vi "rs3_cull_points.vi"(11 "input vertices":dbl[][](array[numeric])=array32964x6[197784 elements]) -> (1 "Valid vertices":bool[](array[boolean]), 2 "output valid vertices":dbl[][](array[numeric]), 3 "Output vertices":string[][](array[string]))   [LabVIEW 2017, in "libRealSense3.lvlib"]
uses:
  libRealSense3.lvlib
panel:
  out "Array 3":bool[](array[boolean])=[FALSE, TRUE, FALSE, TRUE, FALSE, TRUE, FALSE, TRUE, FALSE, TRUE, FALSE, TRUE, FALSE, TRUE, FALSE, TRUE, FALSE, TRUE, FALSE, TRUE, FALSE, TRUE, FALSE, TRUE, FALSE, TRUE, FALSE, TRUE, FALSE, TRUE, FALSE, TRUE, FALSE, TRUE, FALSE, TRUE, FALSE, TRUE, FALSE, TRUE, FALSE, TRUE, FALSE, TRUE, FALSE, TRUE, FALSE, TRUE, FALSE, TRUE, FALSE, TRUE, FALSE, TRUE, FALSE, TRUE, FALSE, TRUE, FALSE, TRUE, FALSE, TRUE, FALSE, TRUE, FALSE, TRUE, FALSE, TRUE, FALSE, TRUE, FALSE, TRUE, FALSE, TRUE, FALSE, TRUE, FALSE, TRUE, FALSE, TRUE, FALSE, TRUE, FALSE, TRUE, FALSE, TRUE, FALSE, TRUE, FALSE, TRUE, FALSE, TRUE, FALSE, TRUE, FALSE, TRUE, FALSE, TRUE, FALSE, TRUE, FALSE, TRUE, FALSE, TRUE, FALSE, TRUE, FALSE, TRUE, FALSE, TRUE, FALSE, TRUE, FALSE, TRUE, FALSE, TRUE, FALSE, TRUE, FALSE, TRUE, FALSE, TRUE, FALSE, TRUE, FALSE, TRUE, FALSE, TRUE, FALSE, TRUE, FALSE, TRUE, FALSE, TRUE, FALSE, TRUE, FALSE, TRUE, FALSE, TRUE, FALSE, TRUE, FALSE, TRUE, FALSE, TRUE, FALSE, TRUE, FALSE, TRUE, FALSE, TRUE, FALSE, TRUE, FALSE, TRUE, FALSE, TRUE, FALSE, TRUE, FALSE, TRUE, FALSE, TRUE, FALSE, TRUE, FALSE, TRUE, FALSE, TRUE, FALSE, TRUE, FALSE, TRUE, FALSE, TRUE, FALSE, TRUE, FALSE, TRUE, FALSE, TRUE, FALSE, TRUE, FALSE, TRUE, FALSE, TRUE, FALSE, TRUE, FALSE, TRUE, FALSE, TRUE, FALSE, TRUE, FALSE, TRUE, FALSE, TRUE, FALSE, TRUE, FALSE, TRUE, FALSE, TRUE, FALSE, TRUE, FALSE, TRUE, FALSE, TRUE, FALSE, TRUE, FALSE, TRUE, FALSE, TRUE, FALSE, TRUE, FALSE, TRUE, FALSE, TRUE, FALSE, TRUE, FALSE, TRUE, FALSE, TRUE, FALSE, TRUE, FALSE, TRUE, FALSE, TRUE, FALSE, TRUE, FALSE, TRUE, FALSE, TRUE, FALSE, TRUE, FALSE, TRUE, FALSE, TRUE, FALSE, TRUE, FALSE, TRUE, FALSE, TRUE, FALSE, TRUE, FALSE, TRUE, FALSE, TRUE, FALSE, TRUE, FALSE, TRUE, FALSE, TRUE, FALSE, TRUE, FALSE, TRUE, FALSE, TRUE, FALSE, TRUE, FALSE, TRUE, FALSE, TRUE, FALSE, TRUE, FALSE, TRUE, FALSE, TRUE, FALSE, TRUE, FALSE, TRUE, FALSE, TRUE, FALSE, TRUE, FALSE, TRUE, FALSE, TRUE, FALSE, TRUE, FALSE, TRUE, FALSE, TRUE, FALSE, TRUE, FALSE, TRUE, FALSE, TRUE, FALSE, TRUE, FALSE, TRUE, FALSE, TRUE, FALSE, TRUE, FALSE, TRUE, FALSE, TRUE, FALSE, TRUE, FALSE, TRUE, FALSE, TRUE, FALSE, TRUE, FALSE, TRUE, FALSE, TRUE, FALSE, TRUE, FALSE, TRUE, FALSE, TRUE, FALSE, TRUE, FALSE, TRUE, FALSE, TRUE, FALSE, TRUE, FALSE, TRUE, FALSE, TRUE, FALSE, TRUE, FALSE, TRUE, FALSE, TRUE, FALSE, TRUE, FALSE, TRUE, FALSE, TRUE, FALSE, TRUE, FALSE, TRUE, FALSE, TRUE, FALSE, TRUE, FALSE, TRUE, FALSE, TRUE, FALSE, TRUE, FALSE, TRUE, FALSE, TRUE, FALSE, TRUE, FALSE, TRUE, FALSE, TRUE, FALSE, TRUE, FALSE, TRUE, FALSE, TRUE, FALSE, TRUE, FALSE, TRUE, FALSE, TRUE, FALSE, TRUE, FALSE, TRUE]
  out "last size":i32=134
  out "last valid":bool=TRUE
  out "Array 2":i32[](array[numeric])=[32, 132, 33, 131, 33, 131, 33, 131, 34, 130, 35, 129, 35, 129, 36, 128, 36, 128, 35, 129, 37, 127, 37, 127, 38, 126, 38, 126, 35, 129, 34, 130, 34, 130, 34, 130, 34, 130, 34, 130, 34, 130, 34, 130, 34, 130, 34, 130, 35, 129, 36, 128, 37, 127, 37, 127, 36, 128, 35, 129, 35, 129, 34, 130, 34, 130, 34, 130, 34, 130, 34, 130, 34, 130, 33, 131, 33, 131, 33, 131, 33, 131, 33, 131, 33, 131, 32, 132, 33, 131, 34, 130, 34, 130, 34, 130, 34, 130, 33, 131, 33, 131, 33, 131, 33, 131, 32, 132, 32, 132, 32, 132, 32, 132, 32, 132, 32, 132, 32, 132, 33, 131, 32, 132, 31, 133, 31, 133, 32, 132, 31, 133, 32, 132, 32, 132, 32, 132, 32, 132, 32, 132, 32, 132, 33, 131, 34, 130, 35, 129, 35, 129, 35, 129, 33, 131, 33, 131, 33, 131, 33, 131, 33, 131, 32, 132, 32, 132, 32, 132, 32, 132, 32, 132, 32, 132, 32, 132, 33, 131, 34, 130, 35, 129, 35, 129, 35, 129, 35, 129, 35, 129, 34, 130, 34, 130, 33, 131, 33, 131, 34, 130, 33, 131, 34, 130, 34, 130, 34, 130, 33, 131, 32, 132, 33, 131, 33, 131, 34, 130, 34, 130, 34, 130, 34, 130, 33, 131, 33, 131, 33, 131, 32, 132, 32, 132, 31, 133, 30, 134, 31, 133, 31, 133, 31, 133, 31, 133, 31, 133, 32, 132, 32, 132, 33, 131, 33, 131, 33, 131, 32, 132, 31, 133, 31, 133, 31, 133, 31, 133, 30, 134, 30, 134, 29, 135, 29, 135, 30, 134, 30, 134, 30, 134, 31, 133, 31, 133, 31, 133, 31, 133, 32, 132, 32, 132, 32, 132, 34, 130, 34, 130, 32, 132, 32, 132, 31, 133, 31, 133, 31, 133, 32, 132, 31, 133, 31, 133, 31, 133, 31, 133, 30, 134, 30, 134, 31, 133, 31, 133, 31, 133, 31, 133, 31, 133, 31, 133, 31, 133, 32, 132, 30, 134, 30, 134, 30, 134, 30, 134, 31, 133, 31, 133, 31, 133, 31, 133, 31, 133, 31, 133, 31, 133, 32, 132, 33, 131, 33, 131, 33, 131, 33, 131, 33, 131, 34, 130, 34, 130, 33, 131, 32, 132, 32, 132, 32, 132, 31, 133, 31, 133, 32, 132, 32, 132, 31, 133, 30, 134, 30, 134]
  out "size(s)":i32[](array[numeric])=[32964, 6]
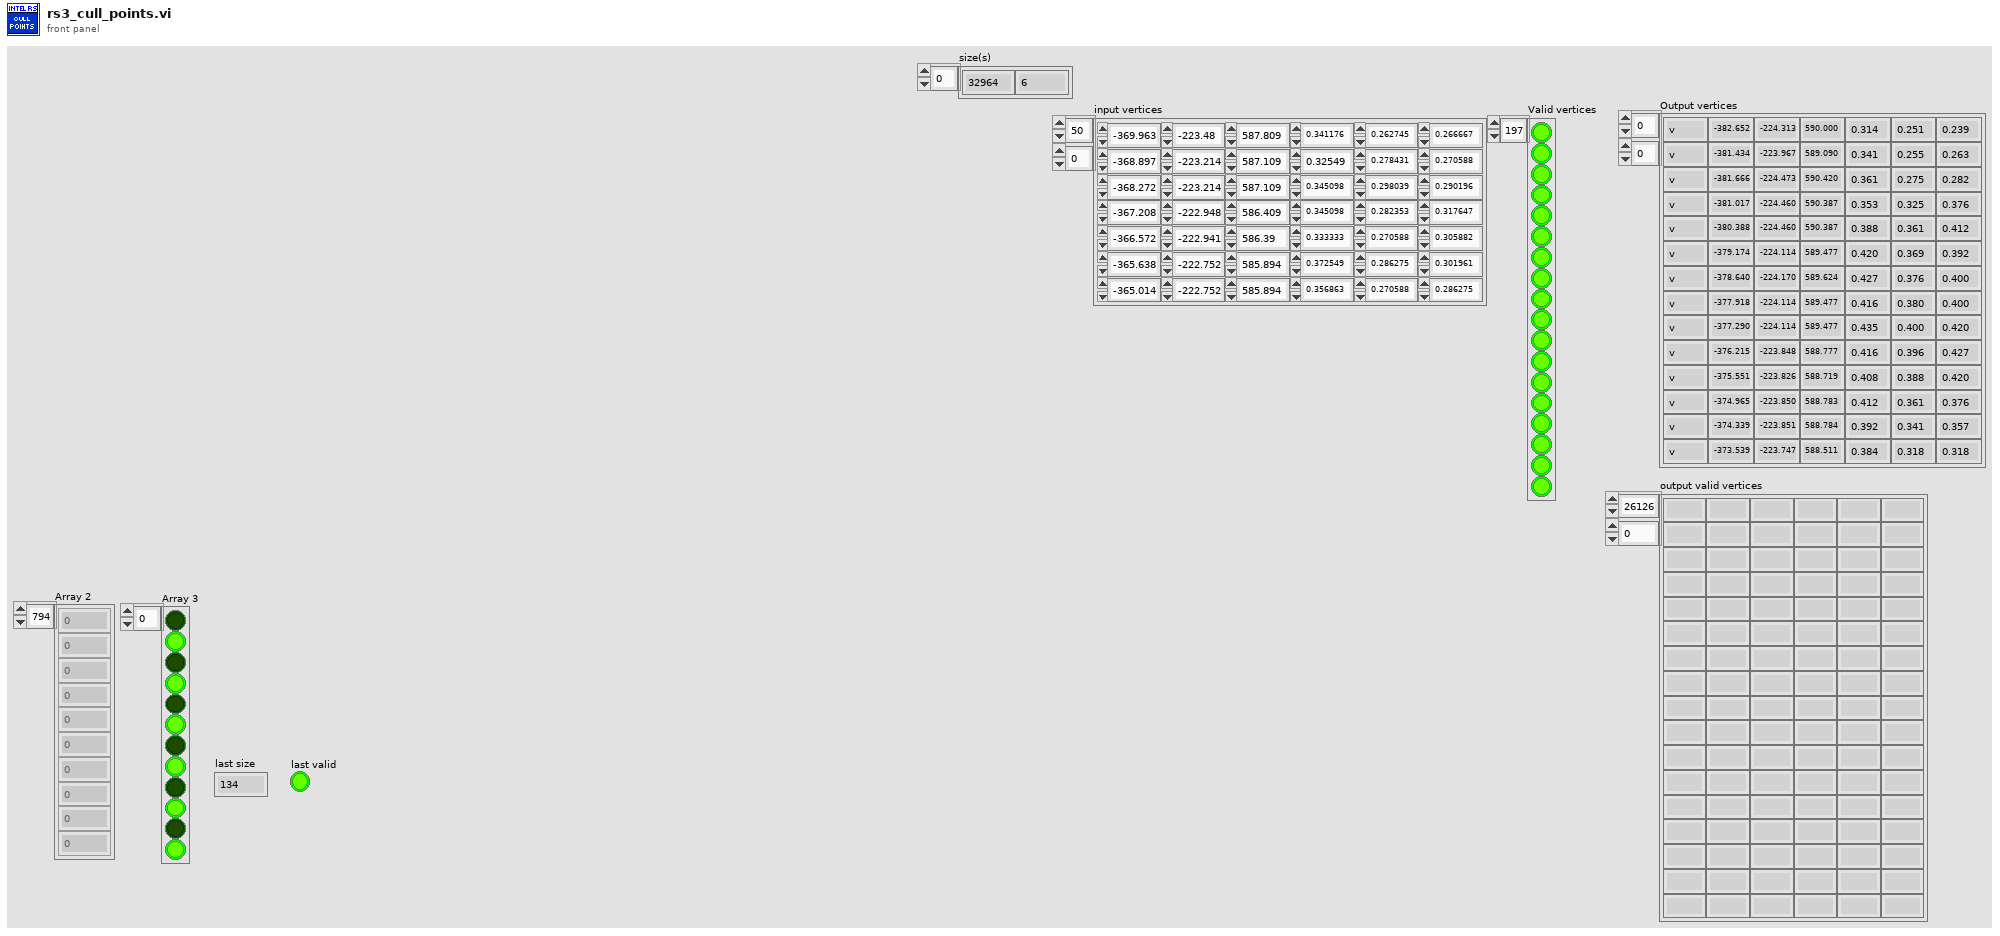
[diagram p1: front panel]
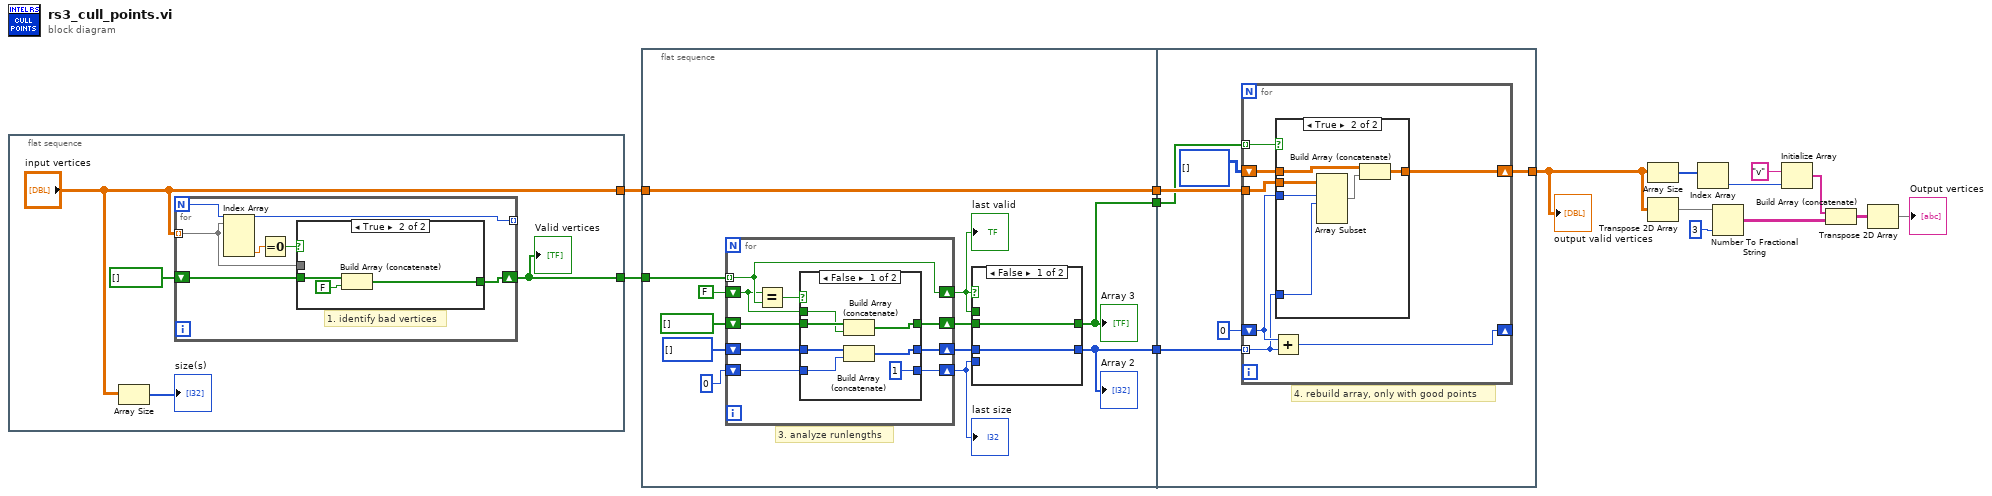
[diagram p0: block diagram]
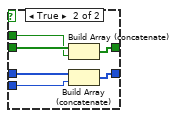
[diagram p2: hidden frame]
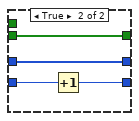
[diagram p3: hidden frame]
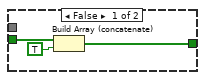
[diagram p5: hidden frame]
diagram:
  n1 = flat-sequence {
    tunnel: [w17] -> w1
    tunnel: ["input vertices"] -> w2
    frame #0 {
      n2 = Array Size(array="input vertices") -> (size(s)=→"size(s)":i32[])
      n3 = for {
        N -> [w23]
        tunnel: "input vertices" -> [w25] mode=indexing
        tunnel: [w23] -> _ mode=indexing
        shift-right: [w21] -> w17
        shift-left: bool[] [] -> [w22]
        # "1. identify bad vertices"
        n4 = Index Array(array=w25) -> (element #3=w20:dbl)  [unwired: 3 in, 2 out]
        n5 = Equal To 0?(x=w20) -> (x = 0?=w24:bool)
        n6 = case shown="True" w24 {
          tunnel: w25 -> [_ _]
          tunnel: [w28 w29] -> w21
          tunnel: w22 -> [w26 w31]
          frame False {
            n7 = Build Array (concatenate)(w26, TRUE) -> (w28:bool[])
          }
          frame True {
            n8 = Build Array (concatenate)(w31, FALSE) -> (w29:bool[])
          }
        }
      }
      "Valid vertices" <- w17
    }
  }
  n9 = flat-sequence {
    tunnel: [w33] -> w5
    tunnel: [w34] -> w4
    tunnel: [w35] -> w3
    tunnel: w2 -> [w33]
    tunnel: w1 -> [w32]
    tunnel: w5 -> [w77]
    tunnel: w4 -> [w74]
    tunnel: w3 -> [w76]
    tunnel: [w72] -> w12
    frame #0 {
      # "3. analyze runlengths"
      n10 = for {
        tunnel: w32 -> [w55] mode=indexing
        shift-right: [w55] -> w38
        shift-left: FALSE -> [w52]
        shift-right: [w59] -> w36
        shift-left: 0 -> [w60]
        shift-right: [w58] -> w37
        shift-left: i32[] [] -> [w57]
        shift-right: [w53] -> w39
        shift-left: bool[] [] -> [w54]
        n11 = Equal?(x=w52, y=w55) -> (x = y?=w56:bool)
        n12 = case shown="False" w56 {
          tunnel: w60 -> [w61 w71]
          tunnel: [1 w70] -> w59
          tunnel: [w66 w69] -> w58
          tunnel: w57 -> [w65 w69]
          tunnel: w54 -> [w64 w68]
          tunnel: [w63 w68] -> w53
          tunnel: w52 -> [w62 _]
          frame False {
            n13 = Build Array (concatenate)(w64, w62) -> (w63:bool[])
            n14 = Build Array (concatenate)(w65, w61) -> (w66:i32[])
          }
          frame True {
            n15 = Increment(x=w71) -> (x+1=w70:i32)
          }
        }
      }
      "last size" <- w36
      "last valid" <- w38
      n16 = case shown="False" w38 {
        tunnel: w39 -> [w45 w51]
        tunnel: w38 -> [_ w50]
        tunnel: w37 -> [w44 w49]
        tunnel: w36 -> [_ w48]
        tunnel: [w44 w47] -> w35
        tunnel: [w45 w46] -> w34
        frame False {
        }
        frame True {
          n17 = Build Array (concatenate)(w51, w50) -> (w46:bool[])
          n18 = Build Array (concatenate)(w49, w48) -> (w47:i32[])
        }
      }
      "Array 3" <- w34
      "Array 2" <- w35
    }
    frame #1 {
      # "4. rebuild array, only with good points"
      n19 = for {
        shift-right: [w82] -> _
        shift-left: 0 -> [w83]
        tunnel: w77 -> [w84]
        tunnel: w76 -> [w81] mode=indexing
        shift-right: [w78] -> w72
        shift-left: i32[][] [] ("all faces input") -> [w80]
        tunnel: w74 -> [w79] mode=indexing
        n20 = Add(x=w83, y=w81) -> (x+y=w82:i32)
        n21 = case shown="True" w79 {
          tunnel: w84 -> [_ w91]
          tunnel: w83 -> [_ w90]
          tunnel: w81 -> [_ w88]
          tunnel: w80 -> [w85 w86]
          tunnel: [w85 w87] -> w78
          frame False {
          }
          frame True {
            n22 = Array Subset(array=w91, index (row)=w90, length (row)=w88) -> (w89:dbl[][])  [unwired: 2 in]
            n23 = Build Array (concatenate)(w86, w89) -> (w87:dbl[][])
          }
        }
      }
    }
  }
  n24 = Array Size(array=w12) -> (size(s)=w14:i32[])
  n25 = Transpose 2D Array(2D array=w12) -> (transposed array=w11:dbl[][])
  n26 = Index Array(array=w14) -> (element=w13:i32)  [unwired: 1 in]
  n27 = Number To Fractional String(number=w11, precision (6)=i16 3) -> (F-format string=w8:string[][])  [unwired: 2 in]
  n28 = Initialize Array("v", w13) -> (w9:string[])
  n29 = Build Array (concatenate)(w9, w8) -> (w7:string[][])
  n30 = Transpose 2D Array(2D array=w7) -> (transposed array=→"Output vertices":string[][])
  "output valid vertices" <- w12
